vi "DB.interpolate_lua.vi"(5 "LuaVIEW reference":T1) -> (15 "error out":errorcluster)   [LabVIEW 2012]
doc: "Interpolate tag values at the specified times. When the tag is a number tag of \"sample\" temporal type, the interpolation is linear between the two points nearest to each time being interpolated at. When the tag is either a numer or a string tag of \"set&hold\" temporal type, interpolation returns the last value logged prior to the specified time since such tags hold their value until changed.\n\nNote that this function tries to read the timerange covered by the specified times from the tag log before commencing with interpolation. This fails when the timerange contains more than \"max points\" points. In such an event, the specified times are divided in increasingly smaller chunks until the reads succeed. In this eventuality, it helps performance when the specified times increase or decrease monitonically.\n\nBeware that this function may take a while to complete. Because of contention this can happen even when the amount of data being queried is small.\nParameters:\nobj:db, database object.\nstr:tag, name of the tag.\ntab:times, timestamps to interpolate at.\nResults:\ntab:values, values interpolated at the given timestamps.\nErrors:\nTag does not exist.\nDatabases module not initialised.\nCannot interpolate more than \"max points\" times in one go.\nCannot interpolate tags of \"event\" temporal type.\nCannot interpolate string tags of \"sample\" temporal type.\nCannot interpolate a timerange containing more than \"max points\" values."
uses:
  luaview/typedefs/t_LuaVIEW Reference.ctl
  luaview/subvis/private/LuaVIEW Pull (string).vi
  luaview/subvis/private/re_LuaVIEW Pull (flat data).vi
  luaview/subvis/private/re_LuaVIEW Push (flat data).vi
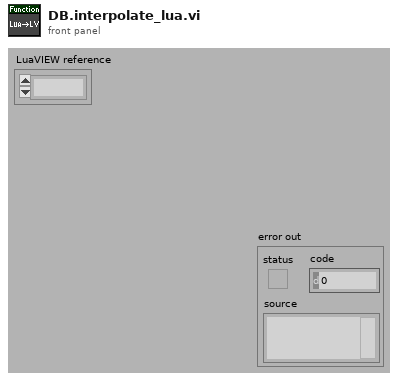
[diagram p1: front panel]
types:
  T1 = typedef "t_LuaVIEW Reference.ctl" = refnum<k1>
  T2 = typedef "t_DataLog Database Info Pane.ctl" = refnum<vi>
  T3 = typedef "t_DataLog Tag Config.ctl" = cluster{"name":string, "unit":string, "temporal":T4, "value":T5, "index":i32, "capacity":i32, "is meta?":bool, "mincapacity":i32, "deadband":dbl, "limit delay":dbl, "format":T6, "precision":u8, "undefine":bool, "update":bool, "update period":u16, "expression":string, "description":string, "logging algorithm":T7, "logging parameters":dbl[]}
  T4 = typedef "t_DataLog Temporal Types.ctl" = enum16{"set&hold", "sample", "event"}
  T5 = typedef "t_DataLog Value Types.ctl" = enum16{"number", "string"}
  T6 = typedef "t_DataLog Numerical Format.ctl" = enum8{"fractional", "exponential", "engineering"}
  T7 = typedef "t_DataLog Logging Algorithms.ctl" = enum16{"nothing", "changes", "everything", "every Nth", "time threshold", "value threshold + prior", "t or v threshold", "t or v threshold + prior"}
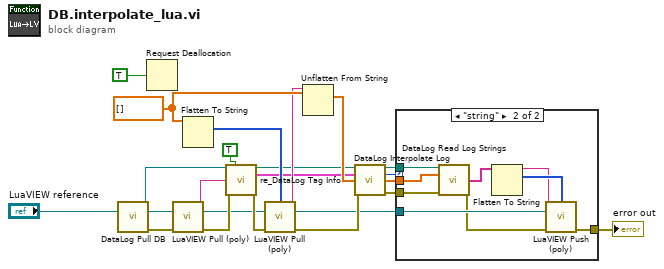
[diagram p0: block diagram]
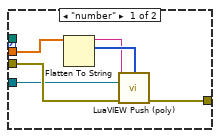
[diagram p2: hidden frame]
diagram:
  w22 = dbl[] [] ("times")
  n1 = call "DataLog Pull DB.vi"("LuaVIEW reference in"="LuaVIEW reference") -> ("database info"=w2:T2, "LuaVIEW reference out"=w4:T1, "error out"=w1:errorcluster)  [unwired: 12 in]
  n2 = Request Deallocation(TRUE ("flag")) -> ()
  n3 = call-poly "LuaVIEW Pull (poly).vi"("LuaVIEW reference in"=w4, "error in (no error)"=w1) -> ("string"=w3:string, "LuaVIEW reference out"=w6:T1, "error out"=w8:errorcluster)  [unwired: 11 in]
  n4 = Flatten To String(anything=w22) -> (type string=w23:i16[])  [unwired: 3 in, 2 out]
  n5 = call "re_DataLog Tag Info.vi"("database ref (use name)"=w2, "flush? (false)"=TRUE, "tag"=w3, "error in (no error)"=w8) -> ("tag log directory"=w10:path, "tag config"=w11:T3, "error out"=w9:errorcluster)  [unwired: 8 in, 1 out]
  n6 = call-poly "LuaVIEW Pull (poly).vi"("type descriptor"=w23, "LuaVIEW reference in"=w6, "error in (no error)"=w9) -> ("flat data"=w21:string, "LuaVIEW reference out"=w18:T1, "error out"=w20:errorcluster)  [unwired: 10 in]
  n7 = Unflatten From String(type=w22, binary string=w21) -> (value=w15:dbl[])  [unwired: 3 in, 2 out]
  n8 = call "DataLog Interpolate Log.vi"("tag log directory"=w10, "tag config"=w11, "times"=w15, "error in (no error)"=w20) -> ("dup tag log directory"=w13:path, "value type"=w16:T5, "interpolated values"=w14:dbl[], "error out"=w19:errorcluster)  [unwired: 8 in]
  n9 = case shown="\"string\"" w16 {
    tunnel: w14 -> [w29 w34]
    tunnel: w19 -> [w28 w32]
    tunnel: w18 -> [w27 w38]
    tunnel: [w24 w35] -> w17
    tunnel: w13 -> [_ w33]
    frame "number" {
      n10 = Flatten To String(anything=w29) -> (data string=w25:string, type string=w26:i16[])  [unwired: 3 in, 1 out]
      n11 = call-poly "LuaVIEW Push (poly).vi"("flat data"=w25, "type descriptor"=w26, "LuaVIEW reference in"=w27, "error in (no error)"=w28) -> ("error out"=w24:errorcluster)  [unwired: 10 in, 1 out]
    }
    frame "string" {
      n12 = call "DataLog Read Log Strings.vi"("tag log directory"=w33, "offsets (use points)"=w34, "error in (no error)"=w32) -> ("strings"=w30:string[], "error out"=w31:errorcluster)  [unwired: 9 in, 2 out]
      n13 = Flatten To String(anything=w30) -> (data string=w36:string, type string=w37:i16[])  [unwired: 3 in, 1 out]
      n14 = call-poly "LuaVIEW Push (poly).vi"("flat data"=w36, "type descriptor"=w37, "LuaVIEW reference in"=w38, "error in (no error)"=w31) -> ("error out"=w35:errorcluster)  [unwired: 10 in, 1 out]
    }
  }
  "error out" <- w17
